vi "KeyenceCVX.Main.Status.vi"(8 "error in":errorcluster, 11 "Data":T1 {"Status"."TriggerNo" items=["1"=1, "2"=2, "3"=3, "4"=4, "ALL"=5]}) -> (0 "error out":errorcluster, 3 "Data out":T1 {"Status"."TriggerNo" items=["1"=1, "2"=2, "3"=3, "4"=4, "ALL"=5]})   [LabVIEW 2016]
uses:
  KeyenceCVX.Data.ctl
  KeyenceCVX.Data.Status.ctl
  KeyenceCVX.Data.Status.State.ctl
  private/controls/TriggerNo.ctl
  private/controls/RunMode.ctl
  KeyenceCVX.Data.Sets.ctl
  KeyenceCVX.CodeDetails.ctl
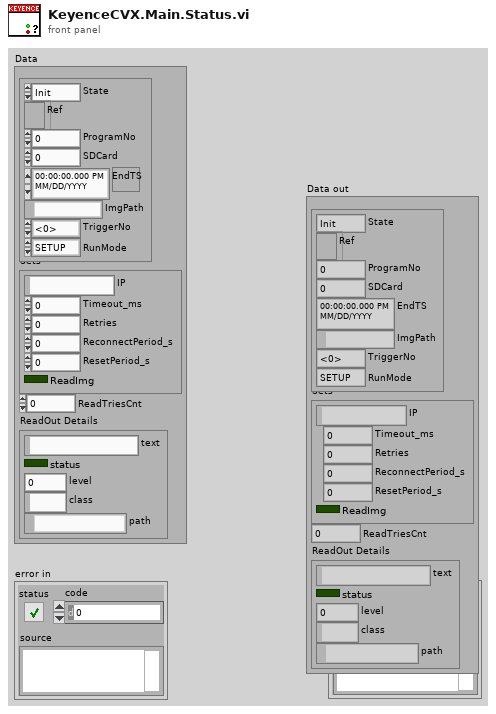
[diagram p1: front panel]
types:
  T1 = typedef "KeyenceCVX.Data.ctl" = cluster{"Status":T2, "Sets":T6, "ReadTriesCnt":u8, "ReadOut Details":T7}
  T2 = typedef "KeyenceCVX.Data.Status.ctl" = cluster{"State":T3, "Ref":refnum<k5>, "ProgramNo":u16, "SDCard":u8, "EndTS":timestamp, "ImgPath":path, "TriggerNo":T4, "RunMode":T5}
  T3 = typedef "KeyenceCVX.Data.Status.State.ctl" = enum16{"Init", "Idle", "Scan", "Reset", "ScanAck", "ChangeProgram"}
  T4 = typedef "TriggerNo.ctl" = u8
  T5 = typedef "RunMode.ctl" = enum16{"SETUP", "RUN"}
  T6 = typedef "KeyenceCVX.Data.Sets.ctl" = cluster{"IP":string, "Timeout_ms":i32, "Retries":i32, "ReconnectPeriod_s":i32, "ResetPeriod_s":i32, "ReadImg":bool}
  T7 = typedef "KeyenceCVX.CodeDetails.ctl" = cluster{"text":string, "status":bool, "level":u8, "class":string, "path":path}
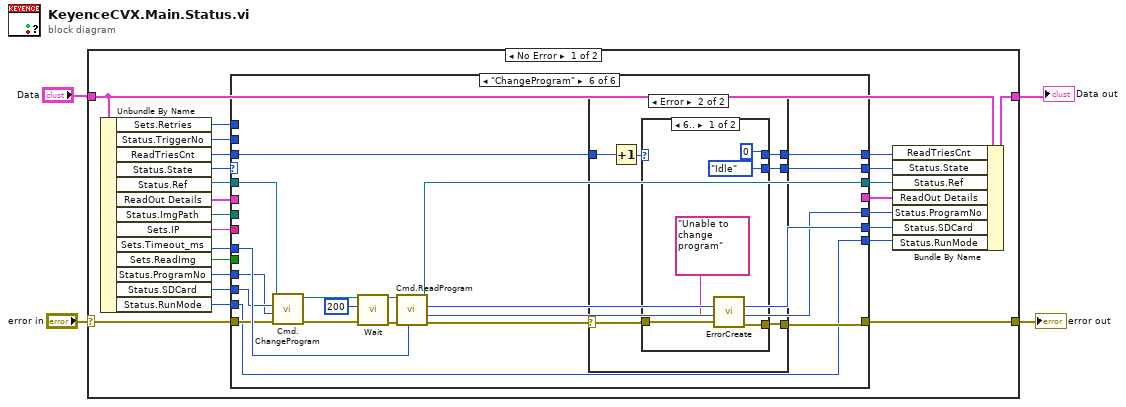
[diagram p0: block diagram]
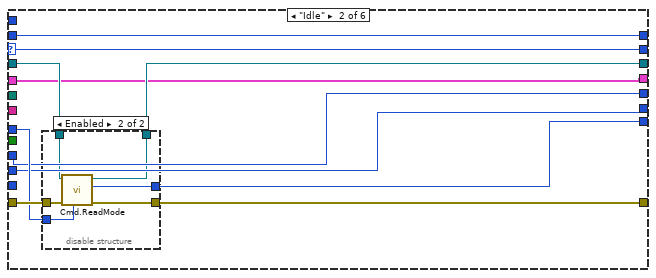
[diagram p3: hidden frame]
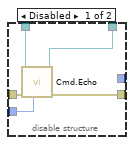
[diagram p4: hidden frame]
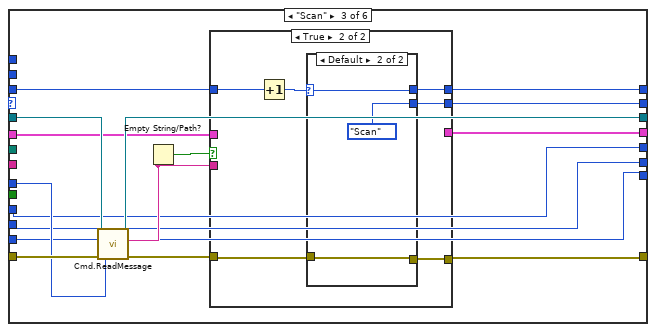
[diagram p5: hidden frame]
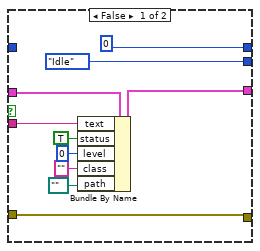
[diagram p6: hidden frame]
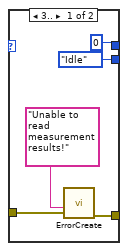
[diagram p7: hidden frame]
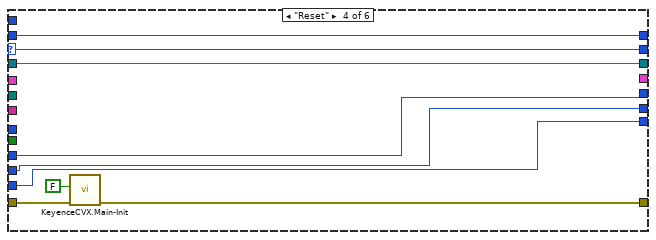
[diagram p8: hidden frame]
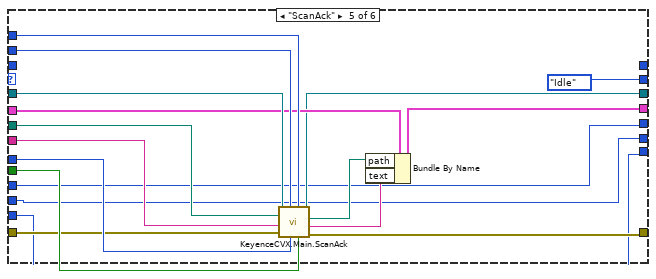
[diagram p9: hidden frame]
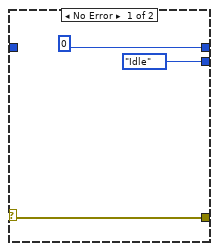
[diagram p10: hidden frame]
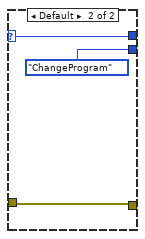
[diagram p11: hidden frame]
diagram:
  n1 = case shown="No Error" "error in" {
    selector: "error in" -> [w26 w162]
    tunnel: [w24 w162] -> w3
    tunnel: "Data" -> [w27 w161]
    tunnel: [w28 w161] -> w1
    frame No Error {
      n2 = Unbundle By Name(w27) -> ("Sets.Retries"=w12:i32, "Status.TriggerNo"=w13:T4, "ReadTriesCnt"=w20:u8, "Status.State"=w25:T3, "Status.Ref"=w23:refnum<k5>, "ReadOut Details"=w17:T7, "Status.ImgPath"=w14:path, "Sets.IP"=w11:string, "Sets.Timeout_ms"=w16:i32, "Sets.ReadImg"=w15:bool, "Status.ProgramNo"=w8:u16, "Status.SDCard"=w7:u8, "Status.RunMode"=w5:T5)
      n3 = case shown="\"ChangeProgram\"" w25 {
        selector: w25 -> [w34 w43 _ w102 _ _]
        tunnel: w26 -> [w36 w47 w74 w106 w123 w134]
        tunnel: [w36 w46 w64 w104 w122 w141] -> w24
        tunnel: w23 -> [w33 w45 w72 w103 w121 w131]
        tunnel: [w33 w44 w71 w103 w112 w137] -> w22
        tunnel: [w34 w43 w70 w102 KeyenceCVX.Data.Status.State."Idle" ("State") w136] -> w21
        tunnel: w20 -> [w35 w42 w69 w107 _ w140]
        tunnel: [w35 w42 w68 w107 _ w139] -> w19
        tunnel: [w32 w41 w67 _ w113 _] -> w18
        tunnel: w17 -> [w32 w41 w62 _ w116 _]
        tunnel: w16 -> [_ w40 w63 _ w125 w142]
        tunnel: w15 -> [_ _ _ _ w124 _]
        tunnel: w14 -> [_ _ _ _ w120 _]
        tunnel: w13 -> [_ _ _ _ w119 _]
        tunnel: w12 -> [_ _ _ _ w118 _]
        tunnel: w11 -> [_ _ _ _ w117 _]
        tunnel: [w30 w38 w60 w100 w109 w135] -> w10
        tunnel: [w31 w39 w61 w101 w110 w128] -> w9
        tunnel: w8 -> [w31 w39 w61 w101 w110 w129]
        tunnel: w7 -> [w30 w38 w60 w100 w109 w132]
        tunnel: [w29 w37 w59 w99 w108 w127] -> w6
        tunnel: w5 -> [w29 _ w59 w99 w108 w127]
        frame Default {
        }
        frame "Idle" {
          n4 = disable-structure shown="Enabled" {
            disable-tunnel: w47 -> [w52 w58]
            disable-tunnel: [w51 w57] -> w46
            disable-tunnel: w45 -> [w50 w55]
            disable-tunnel: [w49 w54] -> w44
            disable-tunnel: w40 -> [w48 w56]
            disable-tunnel: [_ w53] -> w37
            frame Disabled {
              n5 = call "Cmd.Echo.vi"("Timeout [ms] (1000)"=w48, "error in"=w52, "cID in"=w50) -> ("error out"=w51:errorcluster, "cID out"=w49:refnum<k5>)  [unwired: 7 in]
            }
            frame Enabled {
              n6 = call "Cmd.ReadMode.vi"("Timeout [ms] (1000)"=w56, "error in"=w58, "cID in"=w55) -> ("error out"=w57:errorcluster, "RunMode"=w53:T5, "cID out"=w54:refnum<k5>)  [unwired: 6 in]
            }
          }
        }
        frame "Scan" {
          n7 = call "Cmd.ReadMessage.vi"("Timeout [ms] (1000)"=w63, "error in"=w74, "cID in"=w72) -> ("error out"=w65:errorcluster, "Message"=w66:string, "cID out"=w71:refnum<k5>)  [unwired: 6 in]
          n8 = Empty String/Path?(string/path=w66) -> (empty?=w73:bool)
          n9 = case shown="True" w73 {
            tunnel: [KeyenceCVX.Data.Status.State."Idle" ("State") w89] -> w70
            tunnel: w69 -> [_ w90]
            tunnel: [u8 0 w85] -> w68
            tunnel: [w75 _] -> w67
            tunnel: w66 -> [w80 _]
            tunnel: w65 -> [w82 w87]
            tunnel: [w82 w86] -> w64
            tunnel: w62 -> [w81 _]
            frame False {
              n10 = Bundle By Name(cluster=w81, "text"=w80, "status"=TRUE, "level"=u8 0, "class"="", "path"=path "") -> (w75:T7)
            }
            frame True {
              n11 = Increment(x=w90) -> (x+1=w88:u8)
              n12 = case shown="Default" w88 {
                selector: w88 -> [_ w96]
                tunnel: [KeyenceCVX.Data.Status.State."Idle" ("State") KeyenceCVX.Data.Status.State."Scan" ("State")] -> w89
                tunnel: w87 -> [w94 w97]
                tunnel: [w93 w97] -> w86
                tunnel: [u8 0 w96] -> w85
                frame 3.. {
                  n13 = call "ErrorCreate.vi"("error in (no error)"=w94, "ErrorMessage"="Unable to read measurement results!") -> ("error out"=w93:errorcluster)  [unwired: 9 in]
                }
                frame Default {
                }
              }
            }
          }
        }
        frame "Reset" {
          n14 = call "KeyenceCVX.Main-Init.vi"("error in"=w106, "restart (T)"=FALSE) -> ("error out"=w104:errorcluster)  [unwired: 9 in]
        }
        frame "ScanAck" {
          n15 = call "KeyenceCVX.Main.ScanAck.vi"("ReadImg"=w124, "Retries"=w118, "Timeout_ms"=w125, "TriggerNo"=w119, "error in (no error)"=w123, "IP"=w117, "ImgPath"=w120, "TCP Network Connection in"=w121) -> ("error out"=w122:errorcluster, "ReadOut"=w115:string, "File name"=w114:path, "TCP Network Connection out"=w112:refnum<k5>)
          n16 = Bundle By Name(cluster=w116, "path"=w114, "text"=w115) -> (w113:T7)
        }
        frame "ChangeProgram" {
          n17 = call "Cmd.ChangeProgram.vi"("error in"=w134, "Program"=w129, "SDCard"=w132, "cID in"=w131) -> ("error out"=w133:errorcluster, "cID out"=w130:refnum<k5>)  [unwired: 6 in]
          n18 = call "Wait.vi"("error in (no error)"=w133, "Time(ms)"=200) -> ("error out"=w143:errorcluster)  [unwired: 9 in]
          n19 = call "Cmd.ReadProgram.vi"("Timeout [ms] (1000)"=w142, "error in"=w143, "cID in"=w130) -> ("error out"=w126:errorcluster, "ProgramNumber"=w128:u16, "SDCard"=w135:u8, "cID out"=w137:refnum<k5>)  [unwired: 5 in]
          n20 = case shown="Error" w126 {
            selector: w126 -> [w144 w147]
            tunnel: [KeyenceCVX.Data.Status.State."Idle" ("State") w151] -> w136
            tunnel: w140 -> [_ w152]
            tunnel: [u8 0 w148] -> w139
            tunnel: [w144 w149] -> w141
            frame No Error {
            }
            frame Error {
              n21 = Increment(x=w152) -> (x+1=w150:u8)
              n22 = case shown="6.." w150 {
                selector: w150 -> [_ w158]
                tunnel: [KeyenceCVX.Data.Status.State."Idle" ("State") KeyenceCVX.Data.Status.State."ChangeProgram" ("State")] -> w151
                tunnel: w147 -> [w156 w159]
                tunnel: [w155 w159] -> w149
                tunnel: [u8 0 w158] -> w148
                frame 6.. {
                  n23 = call "ErrorCreate.vi"("error in (no error)"=w156, "ErrorMessage"="Unable to change program") -> ("error out"=w155:errorcluster)  [unwired: 9 in]
                }
                frame Default {
                }
              }
            }
          }
        }
      }
      n24 = Bundle By Name(cluster=w27, "ReadTriesCnt"=w19, "Status.State"=w21, "Status.Ref"=w22, "ReadOut Details"=w18, "Status.ProgramNo"=w9, "Status.SDCard"=w10, "Status.RunMode"=w6) -> (w28:T1)
    }
    frame Error {
    }
  }
  "error out" <- w3
  "Data out" <- w1
